vi "FolderMon Organize TDMS.vi"() -> ()   [LabVIEW 2011]
uses:
  DIAdem/lib/DIAdem Daemon Queue.ctl
  DIAdem/lib/DIAdem Daemon Script Type.ctl
  server lib/Spartan Version.vi
  server lib/Spartan CONFIG Global.vi
  Summitek EXT/OpenG EXT/file/file.llb/File Exists - Scalar__ogtk.vi
  Summitek EXT/OpenG EXT/file/file.llb/Convert File Extension (Path)__ogtk.vi
panel:
  out "Files Processed":i32
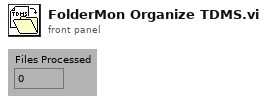
[diagram p1: front panel]
types:
  T1 = typedef "DIAdem Daemon Queue.ctl" = cluster{"Report Template TDM":path, "Report Processor VBS":path, "Report Path PDF":path, "Report Script Params":string, "Username":string, "Script Type":T2, "Report Query Params":string, "Client Machine":string, "Print on Client?":bool, "Response Queue Name":string, "Script Variables":string[], "Start Request Time":timestamp, "Wait?":bool}
  T2 = typedef "DIAdem Daemon Script Type.ctl" = enum16{"Report", "Query", "Script", "Datasheet", "Append", "Restart", "Stop"}
  T3 = enum16{"open", "open or create", "create or replace", "create", "open (read-only)"}
  T4 = typedef "Keyed Array.ctl" = cluster{"keys":string[], "values":string[]}
  T5 = typedef "OGAB Version.ctl" = cluster{"Version":string, "Build Number":u32, "Build Date/Time":dbl}
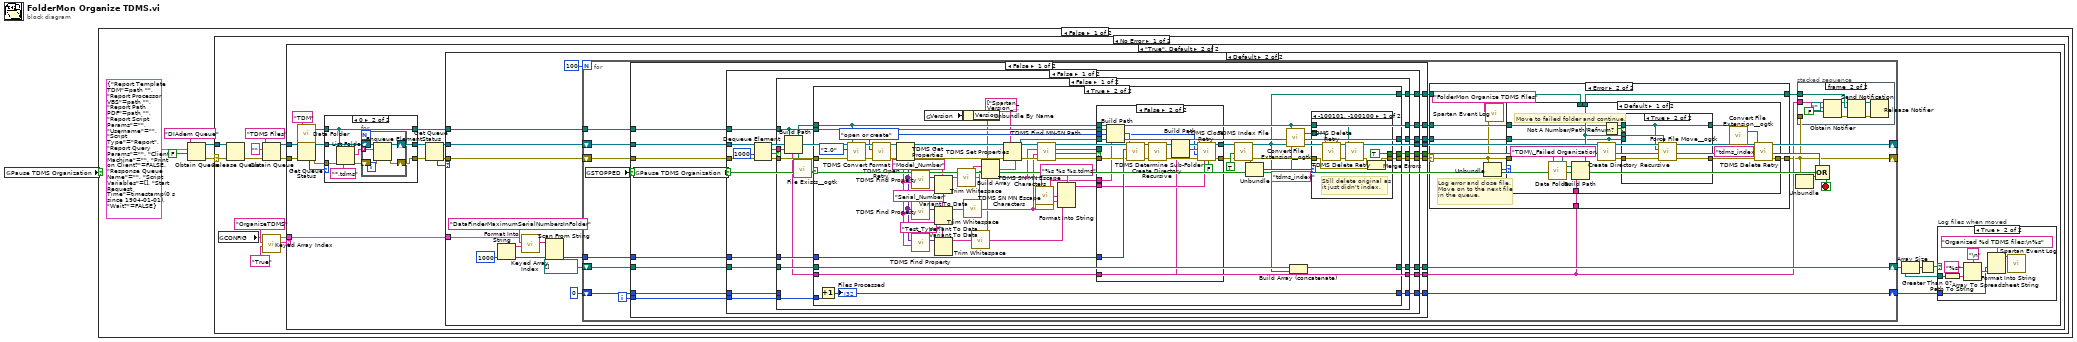
[diagram p0: block diagram]
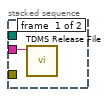
[diagram p5: hidden frame]
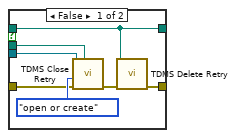
[diagram p7: hidden frame]
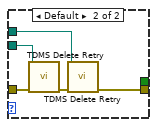
[diagram p10: hidden frame]
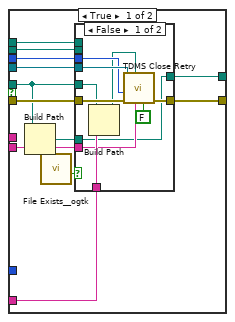
[diagram p11: hidden frame]
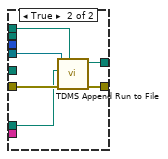
[diagram p12: hidden frame]
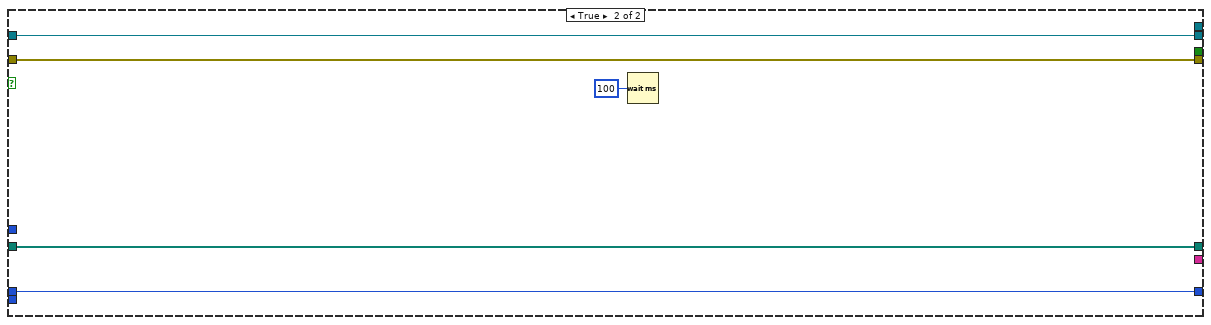
[diagram p14: hidden frame]
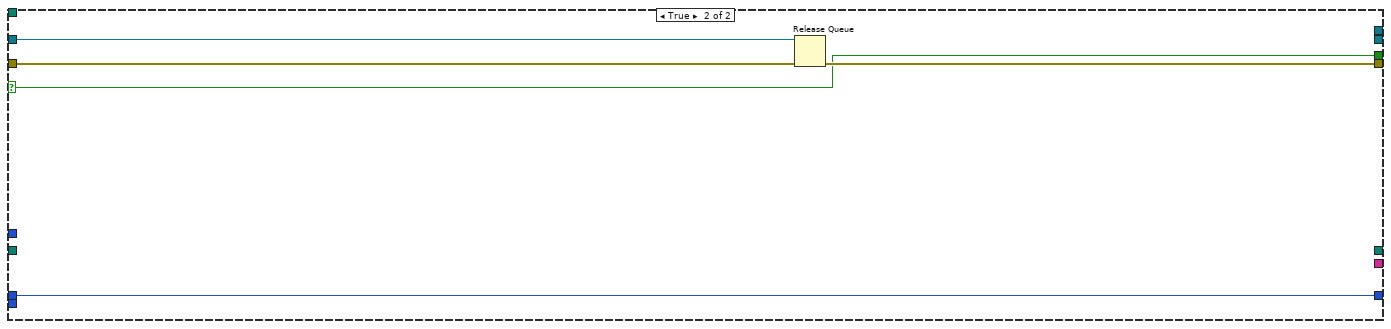
[diagram p15: hidden frame]
diagram:
  n1 = global read "Spartan Version.vi" "Pause TDMS Organization"() -> (w1:bool)
  n2 = case shown="False" w1 {
    frame False {
      n3 = Obtain Queue(name (unnamed)="DIAdem Queue", element data type=T1 {"Report Template TDM"=path "", "Report Processor VBS"=path "", "Report Path PDF"=path "", "Report Script Params"="", "Username"="", "Script Type"=enum."Report", "Report Query Params"="", "Client Machine"="", "Print on Client?"=FALSE, "Response Queue Name"="", "Script Variables"=[], "Start Request Time"=timestamp(0 s since 1904-01-01), "Wait?"=FALSE} ("DD_Report"), create if not found? (T)=FALSE) -> (queue out=w3:refnum<queue>, error out=w4:errorcluster)  [unwired: 2 in, 1 out]
      n4 = case shown="No Error" w4 {
        selector: w4 -> [w9 _]
        tunnel: w3 -> [w7 _]
        frame No Error {
          n5 = global read "Spartan CONFIG Global.vi" "CONFIG"() -> (w13:T4)
          n6 = Release Queue(queue=w7, error in (no error)=w9) -> (error out=w8:errorcluster)  [unwired: 1 in, 2 out]
          n7 = Obtain Queue(name (unnamed)="TDMS Files", element data type="", error in (no error)=w8) -> (queue out=w17:refnum<queue>, error out=w15:errorcluster)  [unwired: 2 in, 1 out]
          n8 = call "Keyed Array Index.vi"("default value"="True", "key"="OrganizeTDMS", "array in"=w13) -> ("value"=w10:string, "duplicate array"=w12:T4)  [unwired: 1 in, 2 out]
          n9 = case shown="\"True\", Default" w10 {
            tunnel: w17 -> [_ w32]
            tunnel: w15 -> [_ w31]
            tunnel: w12 -> [_ w30]
            frame "False" {
            }
            frame "True", Default {
              n10 = call "Data Folder.vi"("Relative Path (\"\" - Folder)"="TDM" ("Relative Path (\"\" - Folder)")) -> ("Data Folder"=w20:path)  [unwired: 2 in]
              n11 = Get Queue Status(queue=w32, error in (no error)=w31) -> (queue out=w26:refnum<queue>, error out=w27:errorcluster, # elements in queue=w21:i32)  [unwired: 1 in, 5 out]
              n12 = case shown="0" w21 {
                tunnel: w26 -> [w33 w42]
                tunnel: [w35 w37] -> w29
                tunnel: w20 -> [w35 w37]
                tunnel: [w34 w39] -> w23
                tunnel: w27 -> [w34 w43]
                tunnel: [w33 w41] -> w25
                frame Default {
                }
                frame 0 {
                  n13 = List Folder(path=w37, pattern="*.tdms", error in=w43) -> (filenames=w36:string[], error out=w40:errorcluster)  [unwired: 1 in, 2 out]
                  n14 = for {
                    shift-right: [w47] -> w39
                    shift-left: w40 -> [w48]
                    tunnel: w36 -> [w45] mode=indexing
                    shift-right: [w44] -> w41
                    shift-left: w42 -> [w46]
                    n15 = Enqueue Element(queue=w46, element=w45, error in (no error)=w48) -> (queue out=w44:refnum<queue>, error out=w47:errorcluster)  [unwired: 1 in, 1 out]
                  }
                }
              }
              n16 = Get Queue Status(queue=w25, error in (no error)=w23) -> (queue out=w24:refnum<queue>, error out=w22:errorcluster, # elements in queue=w19:i32)  [unwired: 1 in, 5 out]
              n17 = case shown="Default" w19 {
                tunnel: w24 -> [_ w60]
                tunnel: w29 -> [_ w61]
                tunnel: w22 -> [_ w54]
                tunnel: w30 -> [_ w53]
                frame 0 {
                }
                frame Default {
                  w56 = 1000
                  n18 = Format Into String(w56) -> (resulting string=w58:string)  [unwired: 3 in, 1 out]
                  n19 = call "Keyed Array Index.vi"("default value"=w58, "key"="DataFinderMaximumSerialNumbersInFolder", "array in"=w53) -> ("value"=w57:string)  [unwired: 1 in, 3 out]
                  n20 = Scan From String(input string=w57, default 1=w56) -> (output 1=w55:i32)  [unwired: 3 in, 3 out]
                  n21 = for {
                    N: 100 -> [_]
                    tunnel: w61 -> [w81]
                    shift-right: [w67] -> _
                    shift-left: w54 -> [w85]
                    tunnel: w55 -> [w84]
                    shift-right: [w82] -> _
                    shift-left: w60 -> [w83]
                    shift-right: [w80] -> w52
                    shift-left: path[] [] -> [w71]
                    shift-right: [w70] -> w49
                    shift-left: 0 -> [w69]
                    i -> [w79]
                    stop <- w76 stop-if-true
                    n22 = global read "Spartan Version.vi" "STOPPED"() -> (w77:bool)
                    n23 = case shown="False" w77 {
                      selector: w77 -> [_ w305]
                      tunnel: w85 -> [w143 w309]
                      tunnel: w84 -> [w148 _]
                      tunnel: w83 -> [w142 w307]
                      tunnel: [w141 _] -> w82
                      tunnel: w81 -> [w147 _]
                      tunnel: [w146 w308] -> w75
                      tunnel: [w145 _] -> w80
                      tunnel: w79 -> [w144 _]
                      tunnel: [w140 w305] -> w78
                      tunnel: [w139 _] -> w74
                      tunnel: [w138 _] -> w73
                      tunnel: w71 -> [w137 _]
                      tunnel: [w136 w306] -> w70
                      tunnel: w69 -> [w135 w306]
                      tunnel: [w134 _] -> w68
                      tunnel: [w133 _] -> w66
                      frame False {
                        n24 = global read "Spartan Version.vi" "Pause TDMS Organization"() -> (w132:bool)
                        n25 = case shown="False" w132 {
                          tunnel: w148 -> [w168 _]
                          tunnel: w147 -> [w167 _]
                          tunnel: [w166 w304] -> w146
                          tunnel: [w165 w301] -> w145
                          tunnel: w144 -> [w164 _]
                          tunnel: w143 -> [w163 w304]
                          tunnel: w142 -> [w161 w303]
                          tunnel: [w160 w303] -> w141
                          tunnel: [w156 _] -> w140
                          tunnel: [w155 _] -> w139
                          tunnel: [w154 _] -> w138
                          tunnel: w137 -> [w153 w301]
                          tunnel: [w152 w302] -> w136
                          tunnel: w135 -> [w151 w302]
                          tunnel: [w150 _] -> w134
                          tunnel: [w149 _] -> w133
                          frame False {
                            n26 = Dequeue Element(queue=w161, timeout in ms (-1)=1000, error in (no error)=w163) -> (queue out=w160:refnum<queue>, element=w159:string, timed out?=w157:bool, error out=w162:errorcluster)
                            n27 = case shown="False" w157 {
                              selector: w157 -> [_ w299]
                              tunnel: w168 -> [w182 _]
                              tunnel: w167 -> [w181 _]
                              tunnel: [w179 w298] -> w166
                              tunnel: [w175 _] -> w165
                              tunnel: w164 -> [w180 _]
                              tunnel: w162 -> [w178 w298]
                              tunnel: w159 -> [w172 _]
                              tunnel: [w173 w299] -> w156
                              tunnel: [w177 _] -> w155
                              tunnel: [w171 _] -> w154
                              tunnel: w153 -> [w176 _]
                              tunnel: [w174 w297] -> w152
                              tunnel: w151 -> [_ w297]
                              tunnel: [w172 _] -> w150
                              tunnel: [w170 _] -> w149
                              frame False {
                                n28 = Build Path(base path=w181, name or relative path=w172) -> (appended path=w171:path)
                                n29 = call-poly "File Exists__ogtk.vi"("file path"=w171) -> ("exists"=w169:bool)  [unwired: 6 in, 1 out]
                                n30 = case shown="True" w169 {
                                tunnel: w182 -> [_ w233]
                                tunnel: w181 -> [_ w230]
                                tunnel: w180 -> [w183 w227]
                                tunnel: [w185 w217] -> w179
                                tunnel: w178 -> [w185 w189]
                                tunnel: [_ w214] -> w177
                                tunnel: w176 -> [w184 w213]
                                tunnel: [w184 w212] -> w175
                                tunnel: [w183 w211] -> w174
                                tunnel: w171 -> [_ w187]
                                tunnel: [_ w209] -> w173
                                tunnel: w172 -> [_ w208]
                                tunnel: [_ w195] -> w170
                                frame False {
                                # "This case can happen if the Queue is empty and the\nfile lister runs at the same time that the save routine\nadds the file to the queue.  The file will get added to\nthe queue twice and this will double check that the file\nhas not already been moved by the organizer before\nproceeding. CHB"
                                }
                                frame True {
                                w232 = "Test_Type" ("Property Name")
                                w234 = "Serial_Number" ("Property Name")
                                w235 = "Model_Number" ("Property Name")
                                w218 = T3."open or create" ("operation (0:open)")
                                n31 = Increment(x=w227) -> (x+1=w211:i32)
                                "Files Processed" <- w211
                                n32 = call <vilib>:"TDMS Convert Format.vi"("error in (no error)"=w189, "target version"=enum16{"1.0", "2.0"}."2.0", "file path"=w187) -> ("error out"=w188:errorcluster, "file path out"=w186:path)  [unwired: 3 in]
                                n33 = call "TDMS Open Retry.vi"("error in (no error)"=w188, "Operation (0:open)"=w218, "Path"=w186) -> ("error out"=w222:errorcluster, "TDMS File Ref"=w221:refnum<k34>)  [unwired: 1 in, 6 out]
                                n34 = TDMS Get Properties(8:w222, 11:w221) -> (0:w216:errorcluster, 3:w219:refnum<k34>, 4:w238:variant[], 6:w239:string[])  [unwired: 4 in, 2 out]
                                n35 = call "TDMS Find Property.vi"("Property Name"=w235, "Property Names"=w239, "Property Values"=w238) -> ("Property Value"=w237:variant)  [unwired: 5 out]
                                n36 = call "TDMS Find Property.vi"("Property Name"=w234, "Property Names"=w239, "Property Values"=w238) -> ("Property Value"=w236:variant)  [unwired: 5 out]
                                n37 = call "TDMS Find Property.vi"("Property Name"=w232, "Property Names"=w239, "Property Values"=w238) -> ("Property Value"=w231:variant)  [unwired: 5 out]
                                n38 = global read "Spartan Version.vi" "Version"() -> (w220:T5)
                                n39 = Variant To Data(type=w235, Variant=w237) -> (data=w207:string)  [unwired: 1 in, 1 out]
                                n40 = Variant To Data(type=w234, Variant=w236) -> (data=w205:string)  [unwired: 1 in, 1 out]
                                n41 = Variant To Data(type=w232, Variant=w231) -> (data=w206:string)  [unwired: 1 in, 1 out]
                                n42 = call <vilib>:"Trim Whitespace.vi"("string"=w207) -> ("trimmed string"=w194:string)  [unwired: 1 in]
                                n43 = Unbundle By Name(w220) -> ("Version"=w204:string)
                                n44 = call <vilib>:"Trim Whitespace.vi"("string"=w205) -> ("trimmed string"=w203:string)  [unwired: 1 in]
                                n45 = call <vilib>:"Trim Whitespace.vi"("string"=w206) -> ("trimmed string"=w202:string)  [unwired: 1 in]
                                n46 = Build Array(w204, w194, w203, w202) -> (w201:string[])
                                n47 = TDMS Set Properties(5:w201, 7:string[] ["Spartan_Version_Current", "Model_Number", "Serial_Number", "Test_Type"], 8:w216, 11:w219) -> (0:w215:errorcluster, 3:w214:refnum<k34>)  [unwired: 2 in, 2 out]
                                n48 = call "TDMS SN MN Escape Characters.vi"("string"=w194) -> ("url-encoded string"=w193:string)
                                n49 = call "TDMS SN MN Escape Characters.vi"("string"=w203) -> ("url-encoded string"=w225:string)
                                n50 = call "TDMS Find MN-SN Path.vi"("error in (no error)"=w215, "Serial Number"=w203, "Model Number"=w194) -> ("error out"=w229:errorcluster, "Found?"=w226:bool, "MN-SN Path"=w228:path)  [unwired: 6 in]
                                n51 = Format Into String(format string="%s %s %s.tdms", w193, w225, w202) -> (resulting string=w223:string)  [unwired: 2 in, 1 out]
                                n52 = case shown="False" w226 {
                                tunnel: w233 -> [_ w296]
                                tunnel: w230 -> [w263 w295]
                                tunnel: w229 -> [w262 w294]
                                tunnel: w193 -> [_ w293]
                                tunnel: w228 -> [w254 _]
                                tunnel: [w261 w288] -> w190
                                tunnel: [w260 w285] -> w191
                                tunnel: w187 -> [w259 _]
                                tunnel: w214 -> [w258 w287]
                                tunnel: w223 -> [w252 w282]
                                tunnel: w218 -> [w255 w283]
                                tunnel: w208 -> [w253 w281]
                                frame True {
                                n53 = Build Path(base path=w254, name or relative path=w252) -> (appended path=w256:path)
                                n54 = call-poly "File Exists__ogtk.vi"("file path"=w256) -> ("exists"=w257:bool)  [unwired: 6 in, 1 out]
                                n55 = case shown="False" w257 {
                                tunnel: w263 -> [_ _]
                                tunnel: w262 -> [w273 w279]
                                tunnel: [w270 w278] -> w261
                                tunnel: [w265 w277] -> w260
                                tunnel: w259 -> [_ w275]
                                tunnel: w258 -> [w272 w276]
                                tunnel: w256 -> [w265 w274]
                                tunnel: w255 -> [w271 _]
                                tunnel: w254 -> [w269 _]
                                tunnel: w253 -> [w268 _]
                                tunnel: w252 -> [w267 _]
                                frame False {
                                n56 = Build Path(base path=w269, name or relative path=w268) -> (appended path=w266:path)
                                n57 = call "TDMS Close Retry.vi"("Release File? (T)"=FALSE, "New TDMS File Name (Optional)"=w267, "TDMS Path"=w266, "error in (no error)"=w273, "Operation (0:open)"=w271, "TDMS File Ref"=w272) -> ("error out"=w270:errorcluster)  [unwired: 3 in, 2 out]
                                }
                                frame True {
                                n58 = call "TDMS Append Run to File.vi"("TDMS Path to Append"=w275, "error in (no error)"=w279, "TDMS Path"=w274, "TDMS File to Append Ref"=w276) -> ("error out"=w278:errorcluster, "TDMS Path"=w277:path)  [unwired: 6 in]
                                }
                                }
                                }
                                frame False {
                                n59 = Build Path(base path=w295, name or relative path=w293) -> (appended path=w289:path)
                                n60 = call "TDMS Determine Sub-Folder.vi"("error in (no error)"=w294, "SN Limit"=w296, "MN Path"=w289) -> ("error out"=w292:errorcluster, "TDMS Path"=w290:path)  [unwired: 7 in]
                                n61 = call <vilib>:"Create Directory Recursive.vi"("error in (no error)"=w292, "directory"=w290) -> ("error out"=w286:errorcluster, "directory copy"=w291:path)  [unwired: 1 in, 3 out]
                                n62 = Build Path(base path=w291, name or relative path=w281) -> (appended path=w284:path)
                                n63 = call "TDMS Close Retry.vi"("Release File? (T)"=FALSE, "New TDMS File Name (Optional)"=w282, "TDMS Path"=w284, "error in (no error)"=w286, "Operation (0:open)"=w283, "TDMS File Ref"=w287) -> ("error out"=w288:errorcluster, "TDMS Path Out"=w285:path)  [unwired: 3 in, 1 out]
                                }
                                }
                                n64 = call "TDMS Index File.vi"("error in (no error)"=w190, "Wait for Index to Complete? (F)"=TRUE, "TDMS File Path"=w191) -> ("error out"=w210:errorcluster, "TDMS File Path Out"=w195:path)  [unwired: 7 in]
                                n65 = Unbundle(w210) -> ("code"=w199:i32)  [unwired: 2 out]
                                n66 = call-poly "Convert File Extension__ogtk.vi"("new ending (none)"="tdms_index", "file name"=w187) -> ("new filename"=w198:path)  [unwired: 1 out]
                                n67 = Build Array (concatenate)(w213, w195) -> (w212:path[])
                                n68 = case shown="-100101, -100100" w199 {
                                tunnel: [w242 w251] -> w217
                                tunnel: w210 -> [w243 w249]
                                tunnel: w187 -> [w245 w248]
                                tunnel: w198 -> [w241 w247]
                                tunnel: [TRUE _] -> w209
                                frame -100101, -100100 {
                                # "Still delete original as\nit just didn't index."
                                n69 = call "TDMS Delete Retry.vi"("path (use dialog)"=w241) -> ("error out"=w246:errorcluster)  [unwired: 10 out]
                                n70 = call "TDMS Delete Retry.vi"("error in"=w246, "path (use dialog)"=w245) -> ("error out"=w244:errorcluster)  [unwired: 9 out]
                                n71 = Merge Errors(w244, w243) -> (w242:errorcluster)
                                }
                                frame Default {
                                n72 = call "TDMS Delete Retry.vi"("error in"=w249, "path (use dialog)"=w247) -> ("error out"=w250:errorcluster)  [unwired: 9 out]
                                n73 = call "TDMS Delete Retry.vi"("error in"=w250, "path (use dialog)"=w248) -> ("error out"=w251:errorcluster)  [unwired: 9 out]
                                }
                                }
                                }
                                }
                              }
                              frame True {
                              }
                            }
                          }
                          frame True {
                            n74 = Wait (ms)(milliseconds to wait=u32 100) -> ()  [unwired: 1 out]
                          }
                        }
                      }
                      frame True {
                        n75 = Release Queue(queue=w307, error in (no error)=w309) -> (error out=w308:errorcluster)  [unwired: 1 in, 2 out]
                      }
                    }
                    n76 = case shown="Error" w75 {
                      selector: w75 -> [w96 w102]
                      tunnel: [w96 w101] -> w67
                      tunnel: w74 -> [_ w100]
                      tunnel: w73 -> [_ w103]
                      tunnel: w68 -> [_ w99]
                      tunnel: w66 -> [w95 w98]
                      tunnel: [w95 w97] -> w65
                      frame No Error {
                      }
                      frame Error {
                        # "Log error and close file.\nMove on to the next file\nin the queue."
                        n77 = Unbundle(w102) -> ("code"=w104:i32)  [unwired: 2 out]
                        n78 = call "Spartan Event Log.vi"("error in (no error)"=w102, "module (\"\")"="FolderMon Organize TDMS Files" ("name (unnamed)")) -> ()  [unwired: 3 in, 4 out]
                        n79 = case shown="Default" w104 {
                          tunnel: [w106 w131] -> w101
                          tunnel: w103 -> [w108 _]
                          tunnel: w102 -> [_ w131]
                          tunnel: w100 -> [w110 _]
                          tunnel: w99 -> [w116 _]
                          tunnel: w98 -> [_ w130]
                          tunnel: [w111 w130] -> w97
                          frame Default {
                            # "Move to failed folder and continue."
                            n80 = call "Data Folder.vi"("Relative Path (\"\" - Folder)"="TDM\\_Failed Organization" ("Relative Path (\"\" - Folder)")) -> ("Data Folder"=w114:path)  [unwired: 2 in]
                            n81 = Build Path(base path=w114, name or relative path=w116) -> (appended path=w111:path)
                            n82 = call <vilib>:"Create Directory Recursive.vi"("directory"=w114) -> ("error out"=w115:errorcluster)  [unwired: 2 in, 4 out]
                            n83 = Not A Number/Path/Refnum?(number/path/refnum=w110) -> (NaN/Path/Refnum?=w109:bool)
                            n84 = case shown="True" w109 {
                              tunnel: [w120 w129] -> w118
                              tunnel: w110 -> [w124 _]
                              tunnel: w115 -> [w123 w128]
                              tunnel: w111 -> [w122 w127]
                              tunnel: w108 -> [w119 w126]
                              tunnel: [w119 w126] -> w107
                              frame False {
                                n85 = call "TDMS Close Retry.vi"("TDMS Path"=w122, "error in (no error)"=w123, "Operation (0:open)"=T3."open or create" ("operation (0:open)"), "TDMS File Ref"=w124) -> ("error out"=w121:errorcluster)  [unwired: 5 in, 2 out]
                                n86 = call "TDMS Delete Retry.vi"("error in"=w121, "path (use dialog)"=w119) -> ("error out"=w120:errorcluster)  [unwired: 9 out]
                              }
                              frame True {
                                n87 = call "Force File Move__ogtk.vi"("error in (no error)"=w128, "source"=w126, "target"=w127) -> ("error out"=w129:errorcluster)  [unwired: 3 in, 1 out]
                              }
                            }
                            n88 = call-poly "Convert File Extension__ogtk.vi"("new ending (none)"="tdms_index", "file name"=w107) -> ("new filename"=w112:path)  [unwired: 1 out]
                            n89 = call "TDMS Delete Retry.vi"("error in"=w118, "path (use dialog)"=w112) -> ("error out"=w106:errorcluster)  [unwired: 9 out]
                          }
                          frame -100101, -100100 {
                          }
                        }
                      }
                    }
                    n90 = Unbundle(w67) -> ("status"=w72:bool)  [unwired: 2 out]
                    n91 = stacked-sequence {
                      tunnel: w68 -> [w86 w94]
                      tunnel: w67 -> [_ _]
                      tunnel: w65 -> [_ w93]
                      frame #0 {
                        n92 = call "TDMS Release File.vi"("Filename"=w86) -> ()  [unwired: 10 in, 1 out]
                      }
                      frame #1 {
                        n93 = Obtain Notifier(name (unnamed)=w94, notification data type=path "", create if not found? (T)=FALSE) -> (notifier out=w92:refnum<notifier>, error out=w89:errorcluster)  [unwired: 1 in, 1 out]
                        n94 = Send Notification(notification=w93, notifier=w92, error in (no error)=w89) -> (notifier out=w91:refnum<notifier>, error out=w87:errorcluster)
                        n95 = Release Notifier(notifier=w91, error in (no error)=w87) -> ()  [unwired: 1 in, 3 out]
                      }
                    }
                    n96 = Compound Arithmetic op=OR(w78, w77, w72) -> (w76:bool)
                  }
                  n97 = Array Size(array=w52) -> (size(s)=w63:i32)
                  n98 = Greater Than 0?(x=w63) -> (x > 0?=w64:bool)
                  n99 = case "Log files when moved" shown="True" w64 {
                    tunnel: w52 -> [_ w311]
                    tunnel: w49 -> [_ w310]
                    frame False {
                    }
                    frame True {
                      n100 = Path To String(path=w311) -> (string=w315:string[])
                      n101 = Array To Spreadsheet String(delimiter (Tab)="\n", array=w315, 3:"%s" ("delimiter (Tab)")) -> (spreadsheet string=w312:string)
                      n102 = Format Into String(format string="Organized %d TDMS files:\n%s" ("name (unnamed)"), w310, w312) -> (resulting string=w316:string)  [unwired: 2 in, 1 out]
                      n103 = call "Spartan Event Log.vi"("message (\"\")"=w316) -> ()  [unwired: 4 in, 4 out]
                    }
                  }
                }
              }
            }
          }
        }
        frame Error {
        }
      }
    }
    frame True {
    }
  }
